vi "channel config test.vi"() -> ()   [LabVIEW 2018]
uses:
  <vilib>/LabVIEW Targets/FPGA/cRIO/shared/nicrio_ModuleControls/nicrio_cRIO-9237_DataRatesRing.ctl
  <vilib>/rvi/Emulation/niFpgaGetClockAttributes.vi
  <vilib>/rvi/Emulation/niFpgaSctlEmulationGetInTimedLoop.vi
  <vilib>/rvi/Emulation/niFpgaEmulationReportErrorSimple.vi
  <vilib>/rvi/eio/common/nirviEmuTemplatePropertySet_noerrors.vi
  <vilib>/rvi/Emulation/niFpgaProcessEmulError.vi
  <vilib>/rvi/eio/common/nirviEmuTemplateMethod_errors.vi
  <vilib>/rvi/interface/RandomDataEmulation/niFpgaRandomDataHandleErrors.vi
  <vilib>/rvi/Memory/Memory_Emulation/nirvimemoryFastEmulation.vi
  <vilib>/rvi/Memory/Memory_Emulation/nirvimemoryEmulation.vi
  <vilib>/rvi/Emulation/niFpgaEmulationIsFPGAContextNoSignature.vi
  <vilib>/rvi/DataTransferAndStorage/Container/Common/niFpgaContainerGetUniqueNameForEmu.vi
  <vilib>/rvi/errors/nirviReportUnexpectedCaseInternalError (U32).vi
  <vilib>/rvi/DataTransferAndStorage/Container/Common/niFpgaContainerExecOnDevCompGetState.vi
  <vilib>/rvi/errors/niFpgaSetErrorForExecOnDevCompSimple.vi
  <vilib>/rvi/eio/common/nirviEmuReportErrorAndStop.vi
  <vilib>/rvi/FIFO/Fifo_Resource/nirvififoEmulationSetSize.vi
  <vilib>/rvi/FIFO/Fifo_Resource/nirviFifoEmulationQueueMgr.vi
  <instcachedir>/0/nirviFifoEmulationQueueMgr_E5CAEC123FF24DC58D834DCA3CDAA9B5.lvgen/nirviFifoEmulationQueueMgr_E5CAEC123FF24DC58D834DCA3CDAA9B5_001.vi
  <vilib>/rvi/FIFO/Fifo_Resource/nirvififoEmulationDetermineInputValidOut.vi
  <vilib>/rvi/FIFO/Fifo_Resource/nirvififoEmulationCreateLock.vi
  <vilib>/rvi/FIFO/Fifo_Resource/nirvififoEmulationObtainLock.vi
  <vilib>/rvi/FIFO/Fifo_Resource/nirvififoEmulationReleaseLock.vi
  <vilib>/rvi/occurrence/nirviWaitOnOccurrenceBase.vi
  <vilib>/rvi/errors/nirviReportUnexpectedCaseInternalError.vi
  <vilib>/Utility/error.llb/Clear Errors.vi
  <vilib>/rvi/Emulation/niFpgaCriticalErrorInLSC.vi
  <vilib>/eio/EIOPropertyNode/EIOPropertyNode.xnode
  <vilib>/eio/EIONode/EIONode.xnode
  <vilib>/rvi/DataTransferAndStorage/Container/XNode/niFpgaContainer.xnode
  <vilib>/rvi/interface/RandomDataEmulation/nirviRandomDataFpgaReadWriteTemplate.vi
  <vilib>/rvi/FIFO/Fifo_Resource/niFpgaFifoEmulationRefIn.vi
  <vilib>/rvi/eio/common/nirviEmuTemplatePropertyGet_errors.vi
  <vilib>/rvi/eio/common/nirviEmuTemplatePropertyGet_noerrors.vi
  <vilib>/rvi/eio/common/nirviEmuTemplatePropertySet_errors.vi
panel:
  in  "Acquisition config":T1(array[cluster])=[{"Channel status"=0.0, "Channel count"=0, "Module active"=FALSE}, {"Channel status"=0.0, "Channel count"=0, "Module active"=FALSE}, {"Channel status"=0.0, "Channel count"=0, "Module active"=FALSE}, {"Channel status"=0.0, "Channel count"=0, "Module active"=FALSE}, {"Channel status"=0.0, "Channel count"=0, "Module active"=FALSE}, {"Channel status"=0.0, "Channel count"=0, "Module active"=FALSE}, {"Channel status"=0.0, "Channel count"=0, "Module active"=FALSE}, {"Channel status"=0.0, "Channel count"=0, "Module active"=FALSE}] {"Channel status" format="%#_14f"}
  in  "Data Rate":T2=1 items=["50.000 kS/s (NI 9237)"=1, "25.000 kS/s (NI 9237)"=2, "16.667 kS/s (NI 9237)"=3, "12.500 kS/s (NI 9237)"=4, "10.000 kS/s (NI 9237)"=5, "8.333 kS/s (NI 9237)"=6, "7.143 kS/s (NI 9237)"=7, "6.250 kS/s (NI 9237)"=8, "5.556 kS/s (NI 9237)"=9, "5.000 kS/s (NI 9237)"=10, "4.545 kS/s (NI 9237)"=11, "4.167 kS/s (NI 9237)"=12, "3.846 kS/s (NI 9237)"=13, "3.571 kS/s (NI 9237)"=14, "3.333 kS/s (NI 9237)"=15, "3.125 kS/s (NI 9237)"=16, "2.941 kS/s (NI 9237)"=17, "2.778 kS/s (NI 9237)"=18, "2.632 kS/s (NI 9237)"=19, "2.500 kS/s (NI 9237)"=20, "2.381 kS/s (NI 9237)"=21, "2.273 kS/s (NI 9237)"=22, "2.174 kS/s (NI 9237)"=23, "2.083 kS/s (NI 9237)"=24, "2.000 kS/s (NI 9237)"=25, "1.923 kS/s (NI 9237)"=26, "1.852 kS/s (NI 9237)"=27, "1.786 kS/s (NI 9237)"=28, "1.724 kS/s (NI 9237)"=29, "1.667 kS/s (NI 9237)"=30, "1.613 kS/s (NI 9237)"=31]
  in  "Exit":bool
  in  "Stop acquire":bool
  out "FIFO Data":sgl[](array[numeric])
  out "loop period (usec)":u32
  in  "Enable FIFO":bool
  in  "Start acquire":bool
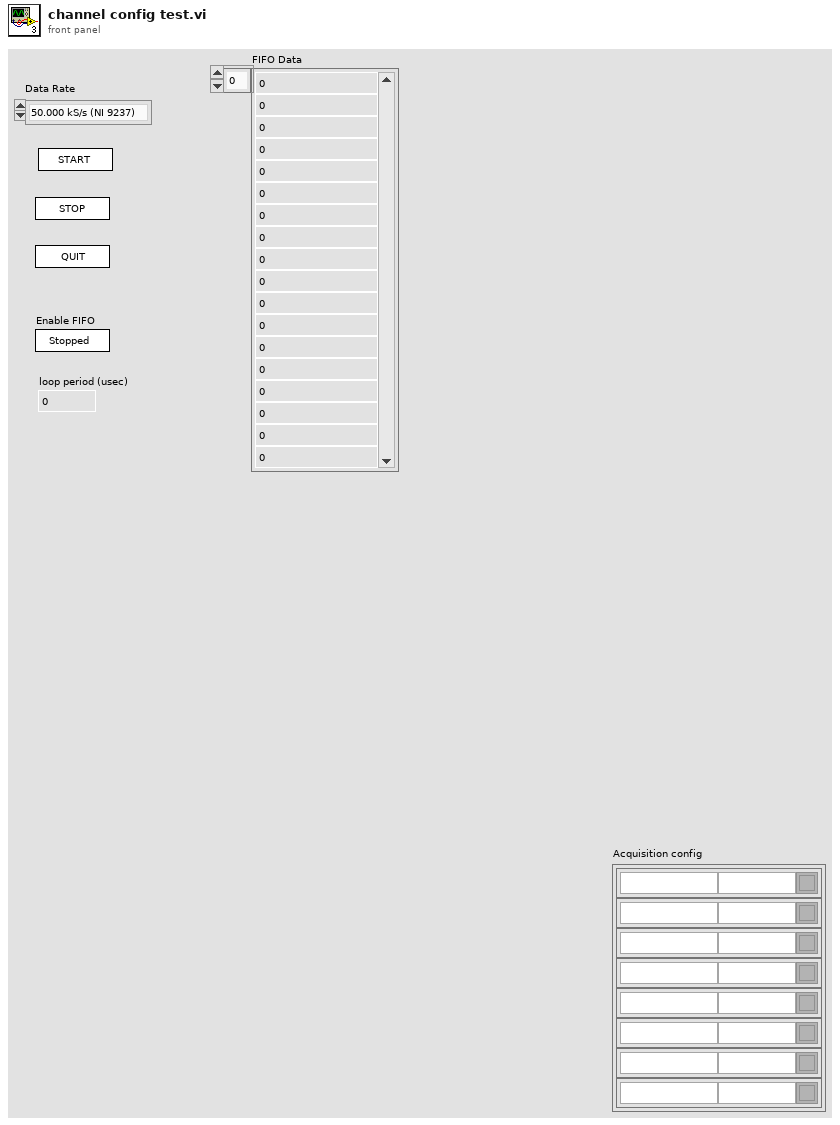
[diagram p1: front panel]
types:
  T1 = cluster{"Channel status":fxp<+,32,32>, "Channel count":u8, "Module active":bool}[]
  T2 = typedef "nicrio_cRIO-9237_DataRatesRing.ctl" = u8
  T3 = cluster{"Active channels":u8[], "Memory offset":i16}[]
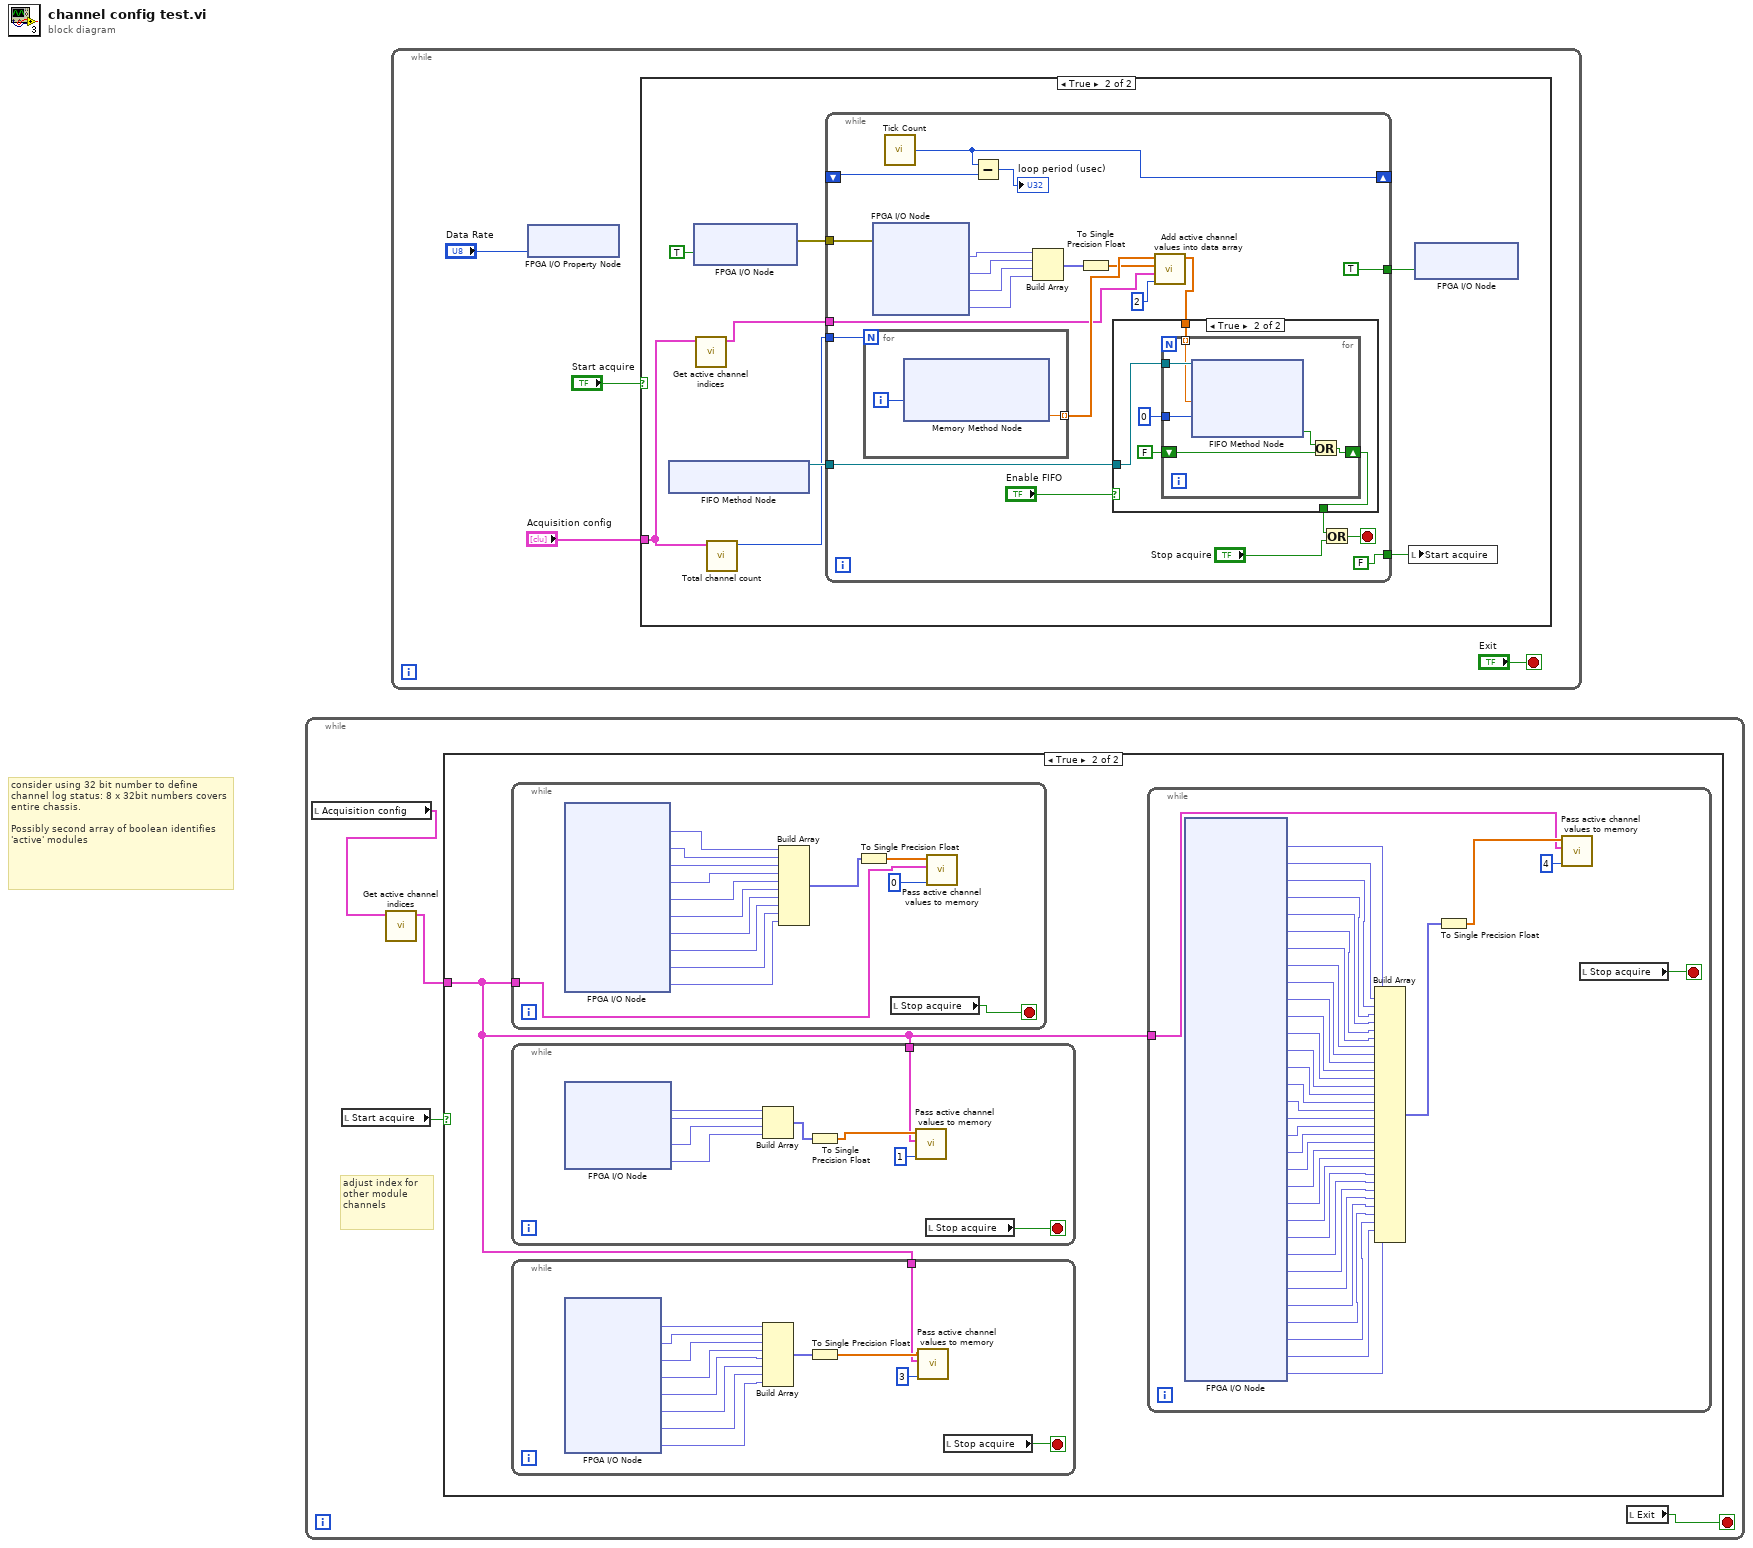
[diagram p0: block diagram]
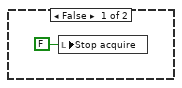
[diagram p3: hidden frame]
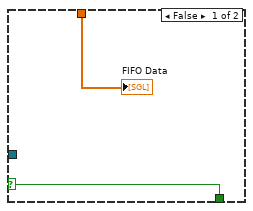
[diagram p4: hidden frame]
diagram:
  # "consider using 32 bit number to define channel log status: 8 x 32bit numbers covers entire chassis.\n\nPossibly second array of boolean identifies 'active' modules"
  n1 = while {
    stop <- w4 stop-if-true
    # "adjust index for other module channels"
    n2 = local read "Acquisition config"() -> (w2:T1)
    n3 = local read "Start acquire"() -> (w3:bool)
    n4 = call "Get active channel indices.vi"("Acquisition config"=w2) -> ("Active channels"=w1:T3)  [unwired: 10 in]
    n5 = case shown="True" w3 {
      tunnel: w1 -> [_ w5]
      frame False {
      }
      frame True {
        n6 = while {
          tunnel: w5 -> [w55]
          stop <- w58 stop-if-true
          n7 = xnode "FPGA I/O Node"() -> ("Mod1/TC0"=w66:fxp<+/-,24,-2>, "Mod1/TC1"=w65:fxp<+/-,24,-2>, "Mod1/TC2"=w64:fxp<+/-,24,-2>, "Mod1/TC3"=w63:fxp<+/-,24,-2>, "Mod1/TC4"=w62:fxp<+/-,24,-2>, "Mod1/TC5"=w61:fxp<+/-,24,-2>, "Mod1/TC6"=w60:fxp<+/-,24,-2>, "Mod1/TC7"=w59:fxp<+/-,24,-2>, "Mod1/CJC0"=w53:fxp<+/-,24,-2>, "Mod1/CJC1"=w52:fxp<+/-,24,-2>)  [unwired: 10 in, 10 out]
          n8 = Build Array(w66, w65, w64, w63, w62, w61, w60, w59, w53, w52) -> (w57:fxp<+/-,24,-2>[])
          n9 = To Single Precision Float(number=w57) -> (single precision float=w56:sgl[])
          n10 = local read "Stop acquire"() -> (w58:bool)
          n11 = call "Pass active channel values to memory.vi"("Module"=0, "Active channels"=w55, "Acquired data"=w56) -> ()  [unwired: 9 in]
        }
        n12 = while {
          tunnel: w5 -> [w44]
          stop <- w46 stop-if-true
          n13 = xnode "FPGA I/O Node"() -> ("Mod2/RTD0"=w51:fxp<+/-,24,10>, "Mod2/RTD1"=w50:fxp<+/-,24,10>, "Mod2/RTD2"=w49:fxp<+/-,24,10>, "Mod2/RTD3"=w47:fxp<+/-,24,10>)  [unwired: 4 in, 4 out]
          n14 = Build Array(w51, w50, w49, w47) -> (w48:fxp<+/-,24,10>[])
          n15 = To Single Precision Float(number=w48) -> (single precision float=w45:sgl[])
          n16 = call "Pass active channel values to memory.vi"("Module"=1, "Active channels"=w44, "Acquired data"=w45) -> ()  [unwired: 9 in]
          n17 = local read "Stop acquire"() -> (w46:bool)
        }
        n18 = while {
          tunnel: w5 -> [w68]
          stop <- w70 stop-if-true
          n19 = xnode "FPGA I/O Node"() -> ("Mod4/AI0"=w79:fxp<+/-,21,-4>, "Mod4/AI1"=w78:fxp<+/-,21,-4>, "Mod4/AI2"=w77:fxp<+/-,21,-4>, "Mod4/AI3"=w75:fxp<+/-,21,-4>, "Mod4/AI4"=w74:fxp<+/-,21,-4>, "Mod4/AI5"=w73:fxp<+/-,21,-4>, "Mod4/AI6"=w72:fxp<+/-,21,-4>, "Mod4/AI7"=w71:fxp<+/-,21,-4>)  [unwired: 8 in, 8 out]
          n20 = Build Array(w79, w78, w77, w75, w74, w73, w72, w71) -> (w76:fxp<+/-,21,-4>[])
          n21 = To Single Precision Float(number=w76) -> (single precision float=w69:sgl[])
          n22 = call "Pass active channel values to memory.vi"("Module"=3, "Active channels"=w68, "Acquired data"=w69) -> ()  [unwired: 9 in]
          n23 = local read "Stop acquire"() -> (w70:bool)
        }
        n24 = while {
          tunnel: w5 -> [w7]
          stop <- w41 stop-if-true
          n25 = xnode "FPGA I/O Node"() -> ("Mod5/AI0"=w9:fxp<+/-,26,5>, "Mod5/AI1"=w10:fxp<+/-,26,5>, "Mod5/AI2"=w11:fxp<+/-,26,5>, "Mod5/AI3"=w12:fxp<+/-,26,5>, "Mod5/AI4"=w13:fxp<+/-,26,5>, "Mod5/AI5"=w14:fxp<+/-,26,5>, "Mod5/AI6"=w15:fxp<+/-,26,5>, "Mod5/AI7"=w16:fxp<+/-,26,5>, "Mod5/AI8"=w40:fxp<+/-,26,5>, "Mod5/AI9"=w39:fxp<+/-,26,5>, "Mod5/AI10"=w38:fxp<+/-,26,5>, "Mod5/AI11"=w37:fxp<+/-,26,5>, "Mod5/AI12"=w36:fxp<+/-,26,5>, "Mod5/AI13"=w35:fxp<+/-,26,5>, "Mod5/AI14"=w34:fxp<+/-,26,5>, "Mod5/AI15"=w33:fxp<+/-,26,5>, "Mod5/AI16"=w32:fxp<+/-,26,5>, "Mod5/AI17"=w31:fxp<+/-,26,5>, "Mod5/AI18"=w30:fxp<+/-,26,5>, "Mod5/AI19"=w29:fxp<+/-,26,5>, "Mod5/AI20"=w28:fxp<+/-,26,5>, "Mod5/AI21"=w27:fxp<+/-,26,5>, "Mod5/AI22"=w26:fxp<+/-,26,5>, "Mod5/AI23"=w25:fxp<+/-,26,5>, "Mod5/AI24"=w24:fxp<+/-,26,5>, "Mod5/AI25"=w23:fxp<+/-,26,5>, "Mod5/AI26"=w22:fxp<+/-,26,5>, "Mod5/AI27"=w21:fxp<+/-,26,5>, "Mod5/AI28"=w20:fxp<+/-,26,5>, "Mod5/AI29"=w19:fxp<+/-,26,5>, "Mod5/AI30"=w18:fxp<+/-,26,5>, "Mod5/AI31"=w17:fxp<+/-,26,5>)  [unwired: 32 in, 32 out]
          n26 = Build Array(w9, w10, w11, w12, w13, w14, w15, w16, w40, w39, w38, w37, w36, w35, w34, w33, w32, w31, w30, w29, w28, w27, w26, w25, w24, w23, w22, w21, w20, w19, w18, w17) -> (w42:fxp<+/-,26,5>[])
          n27 = To Single Precision Float(number=w42) -> (single precision float=w8:sgl[])
          n28 = call "Pass active channel values to memory.vi"("Module"=4, "Active channels"=w7, "Acquired data"=w8) -> ()  [unwired: 9 in]
          n29 = local read "Stop acquire"() -> (w41:bool)
        }
      }
    }
    n30 = local read "Exit"() -> (w4:bool)
  }
  n31 = while {
    stop <- "Exit" stop-if-true
    n32 = xnode "FPGA I/O Property Node"("Data Rate"="Data Rate") -> ()  [unwired: 1 in, 1 out]
    n33 = case shown="True" "Start acquire" {
      tunnel: "Acquisition config" -> [_ w86]
      frame False {
        n34 = local write "Stop acquire"(FALSE ("Stop acquire")) -> ()
      }
      frame True {
        n35 = xnode ("FIFO Method Node")() -> ("FIFO Out"=w88:refnum<k21>)  [unwired: 1 in]
        n36 = xnode "FPGA I/O Node"("Mod3/Start"=TRUE) -> ("error out"=w90:errorcluster)  [unwired: 2 in, 1 out]
        n37 = call "Get active channel indices.vi"("Acquisition config"=w86) -> ("Active channels"=w85:T3)  [unwired: 10 in]
        n38 = call "Total channel count.vi"("Acquisition config"=w86) -> ("Total channels"=w87:u8)  [unwired: 10 in]
        n39 = while {
          tunnel: [TRUE ("I/O Item")] -> w91
          tunnel: w90 -> [w113]
          tunnel: w87 -> [w104]
          tunnel: [FALSE] -> w89
          shift-right: [w102] -> _
          shift-left: _ -> [w101]
          tunnel: w88 -> [w98]
          tunnel: w85 -> [w93]
          stop <- w106 stop-if-true
          n40 = for {
            N: w104 -> [_]
            tunnel: [w128] -> w97 mode=indexing
            i -> [w129]
            n41 = xnode ("Memory Method Node")("Address"=w129) -> ("Data"=w128:sgl)  [unwired: 1 in, 1 out]
          }
          n42 = xnode "FPGA I/O Node"("error in"=w113) -> ("Mod3/AI0"=w112:fxp<+/-,24,-4>, "Mod3/AI1"=w111:fxp<+/-,24,-4>, "Mod3/AI2"=w110:fxp<+/-,24,-4>, "Mod3/AI3"=w109:fxp<+/-,24,-4>)  [unwired: 4 in, 5 out]
          n43 = call "Tick Count"() -> ("Tick Count(uSec)"=w102:u32)
          n44 = Subtract(x=w102, y=w101) -> (x-y=→"loop period (usec)":u32)
          n45 = Build Array(w112, w111, w110, w109) -> (w108:fxp<+/-,24,-4>[])
          n46 = To Single Precision Float(number=w108) -> (single precision float=w96:sgl[])
          n47 = call "Add active channel values into data array.vi"("Module"=2, "Active channels"=w93, "Acquired data"=w96, "Memory data"=w97) -> ("Updated data"=w94:sgl[])  [unwired: 7 in]
          n48 = case shown="True" "Enable FIFO" {
            selector: "Enable FIFO" -> [w116 _]
            tunnel: [w116 w120] -> w105
            tunnel: w98 -> [_ w118]
            tunnel: w94 -> [w115 w117]
            frame False {
              "FIFO Data" <- w115
            }
            frame True {
              n49 = for {
                tunnel: 0 ("Timeout") -> [w127]
                shift-right: [w125] -> w120
                shift-left: FALSE -> [w124]
                tunnel: w118 -> [w123]
                tunnel: w117 -> [w122] mode=indexing
                n50 = xnode ("FIFO Method Node")("Element"=w122, "Timeout"=w127, "FIFO In"=w123) -> ("Timed Out?"=w126:bool)  [unwired: 1 out]
                n51 = Or(x=w126, y=w124) -> (x .or. y?=w125:bool)
              }
            }
          }
          n52 = Or(x=w105, y="Stop acquire") -> (x .or. y?=w106:bool)
        }
        n53 = local write "Start acquire"(w89) -> ()
        n54 = xnode "FPGA I/O Node"("Mod3/Stop"=w91) -> ()  [unwired: 1 in, 1 out]
      }
    }
  }
